vi "Continue Z Scan.vi"(7 "Error Signal Notifier":refnum<notifier>, 8 "error in (no error)":errorcluster, 9 "Automation State In":T1, 10 "Automation Queue":refnum<queue>, 11 "UI Queue":refnum<queue>) -> (0 "error out":errorcluster, 1 "Automation State Out":T1, 2 "Keep looping?":bool)   [LabVIEW 2013, in "Automation.lvlib"]
uses:
  Automation.lvlib
  Automation State.ctl
  Zscan Settings.ctl
  support/Message Queue/Message Cluster.ctl
  Feedback/Error Signal.ctl
  support/Message Queue/Enqueue Message (Single).vi
  support/Message Queue/Message Queue.lvlib
  Feedback/Feedback.lvlib
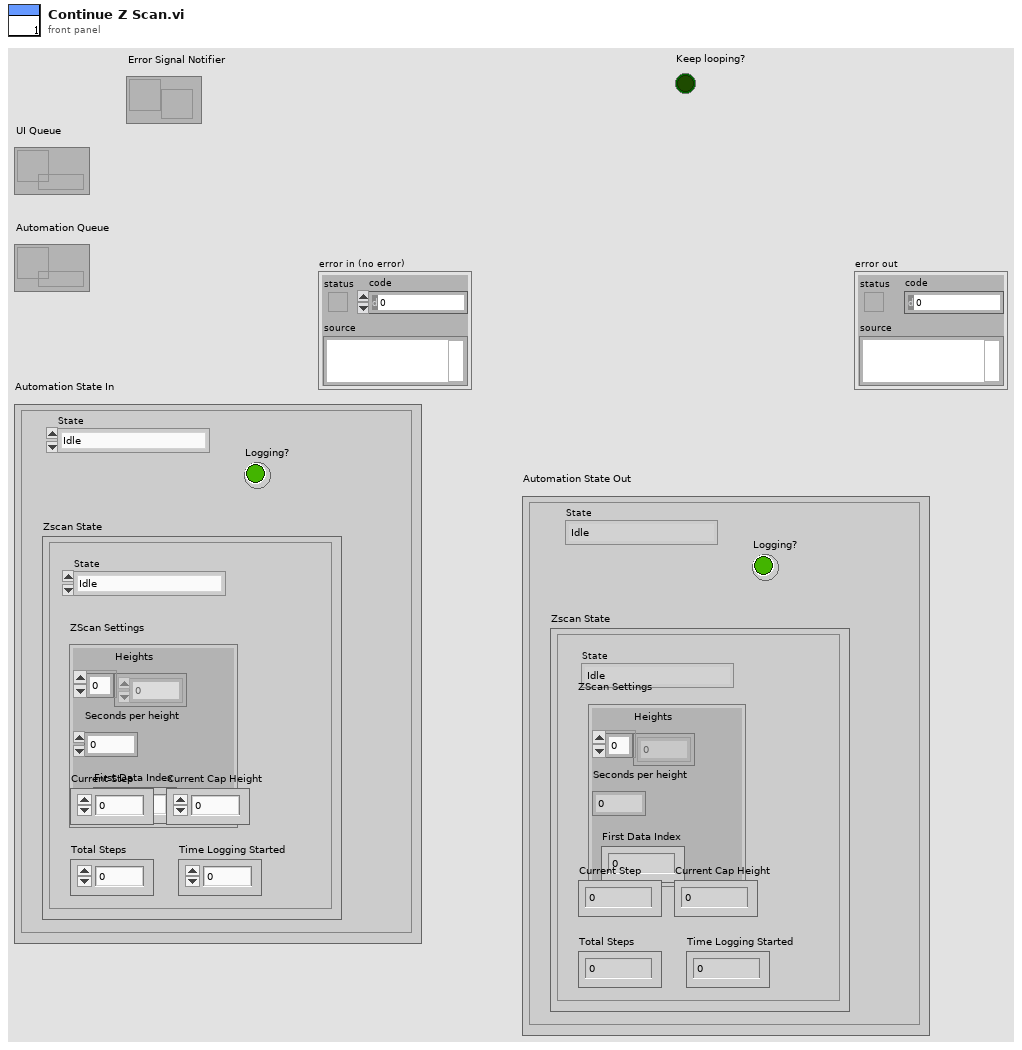
[diagram p1: front panel]
types:
  T1 = typedef "Automation.lvlib/Automation State.ctl" = cluster{"State":enum16{"Idle", "Zscan"}, "Logging?":bool, "Zscan State":cluster{"State":enum16{"Idle", "Waiting for lock", "Waiting for acquisition"}, "ZScan Settings":T2, "Current Step":i32, "Current Cap Height":dbl, "Total Steps":i32, "Time Logging Started":dbl}}
  T2 = typedef "Automation.lvlib/Zscan Settings.ctl" = cluster{"Heights":dbl[], "Seconds per height":i32, "First Data Index":i32}
  T3 = cluster{"State":enum16{"Idle", "Waiting for lock", "Waiting for acquisition"}, "ZScan Settings":T2, "Current Step":i32, "Current Cap Height":dbl, "Total Steps":i32, "Time Logging Started":dbl}
  T4 = enum16{"Idle", "Waiting for lock", "Waiting for acquisition"}
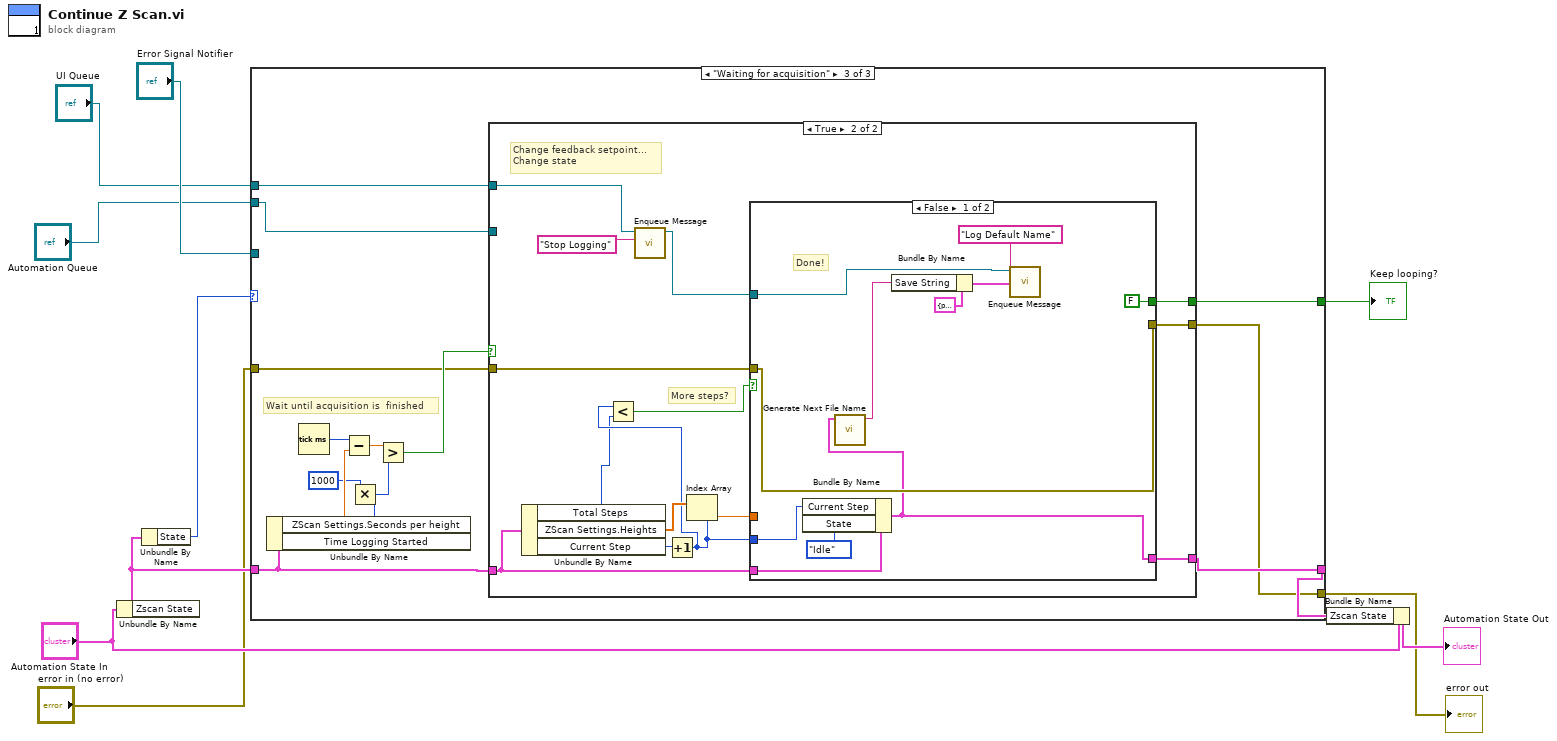
[diagram p0: block diagram]
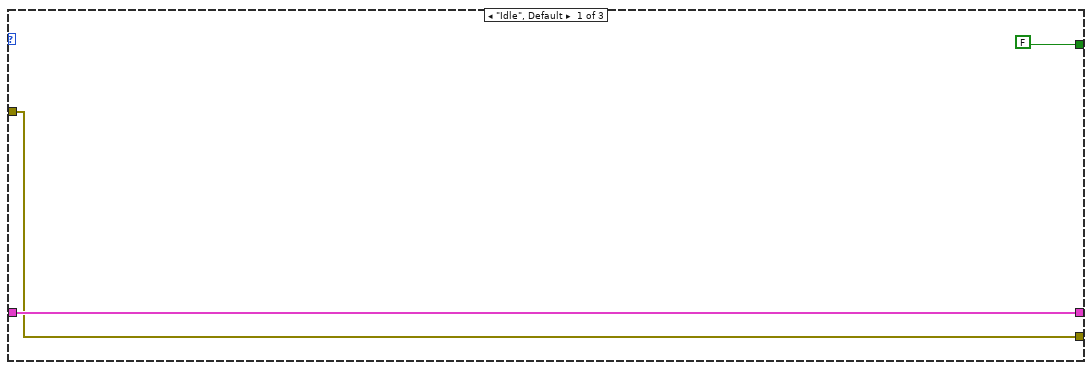
[diagram p2: hidden frame]
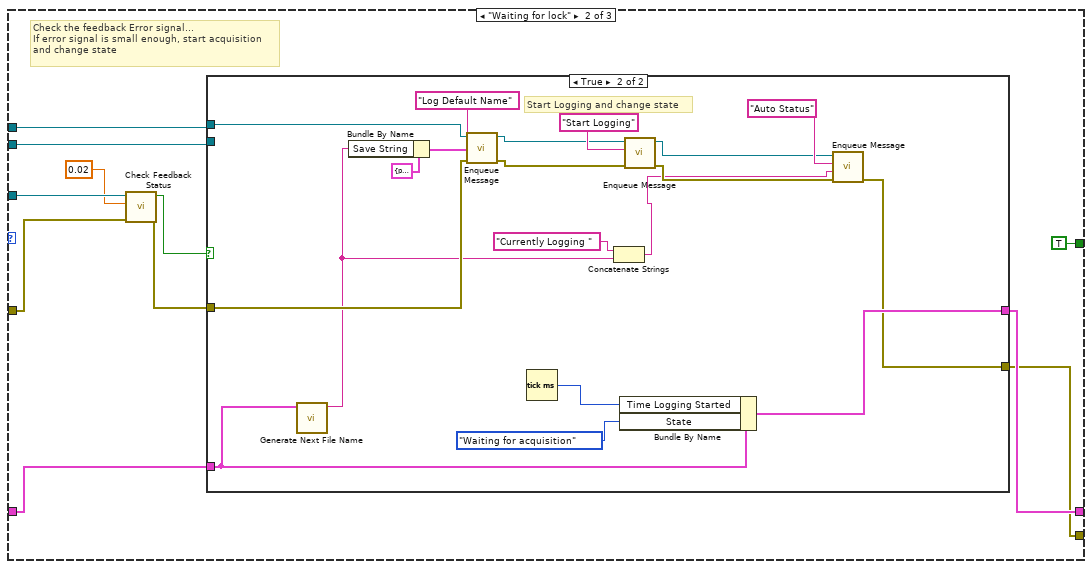
[diagram p3: hidden frame]
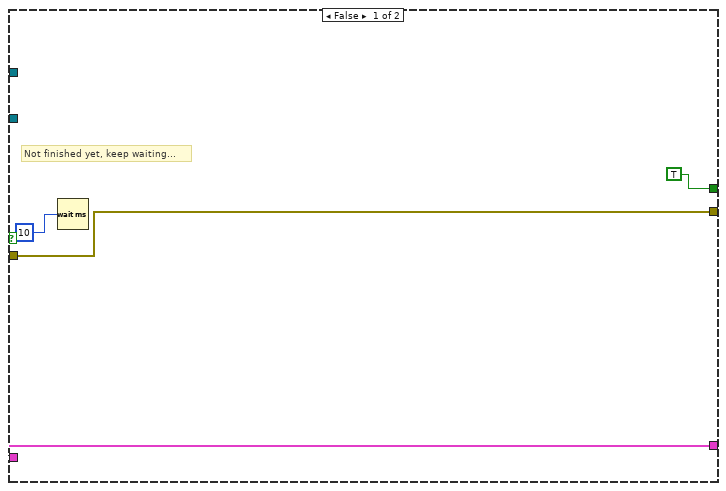
[diagram p5: hidden frame]
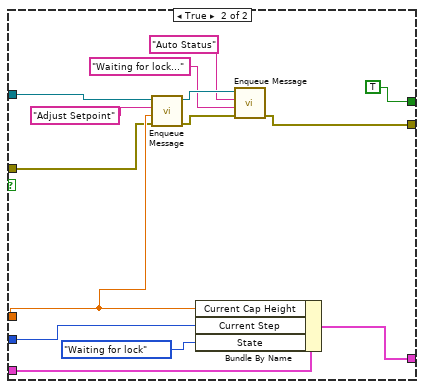
[diagram p6: hidden frame]
diagram:
  n1 = Unbundle By Name("Automation State In") -> ("Zscan State"=w8:T3)
  n2 = Unbundle By Name(w8) -> ("State"=w7:T4)
  n3 = case shown="\"Waiting for acquisition\"" w7 {
    tunnel: [w14 w21 w52] -> w9
    tunnel: w8 -> [w14 w22 w53]
    tunnel: "Error Signal Notifier" -> [_ w25 _]
    tunnel: "Automation Queue" -> [_ w20 w48]
    tunnel: "error in (no error)" -> [w13 w16 w50]
    tunnel: [w13 w19 w49] -> w3
    tunnel: "UI Queue" -> [_ w17 w51]
    tunnel: [FALSE ("Keep looping?") TRUE ("Keep looping?") w47] -> w1
    frame "Idle", Default {
    }
    frame "Waiting for lock" {
      # "Check the feedback Error signal...\nIf error signal is small enough, start acquisition\nand change state"
      n4 = call "Check Feedback Status.vi"("error in (no error)"=w16, "Threshold (um)"=0.02, "Error Signal Notifier"=w25) -> ("error out"=w15:errorcluster, "Locked"=w23:bool)  [unwired: 7 in]
      n5 = case shown="True" w23 {
        tunnel: w22 -> [w27 w32]
        tunnel: [w27 w46] -> w21
        tunnel: w20 -> [_ _]
        tunnel: w15 -> [w26 w35]
        tunnel: [w26 w40] -> w19
        tunnel: w17 -> [_ w28]
        frame False {
          # "If not locked, keep looping"
        }
        frame True {
          # "Start Logging and change state"
          n6 = call "Generate Next File Name.vi"("Zscan State"=w32) -> ("String"=w30:string)  [unwired: 10 in]
          n7 = Bundle By Name(cluster=cluster{"Save Path":path, "Save String":string} {"Save Path"=path "", "Save String"=""} ("output cluster"), "Save String"=w30) -> (w33:cluster{"Save Path":path, "Save String":string})
          n8 = call-poly "Enqueue Message.vi"("error in (no error)"=w35, "Message Data"=w33, "Message"="Log Default Name", "Message Queue"=w28) -> ("error out"=w37:errorcluster, "dup Message Queue"=w36:refnum<queue>)  [unwired: 6 in]
          n9 = Tick Count (ms)() -> (millisecond timer value=w43:u32)
          n10 = Concatenate Strings("Currently Logging " ("Message"), w30) -> (w29:string)
          n11 = Bundle By Name(cluster=w32, "Time Logging Started"=w43, "State"=T4."Waiting for acquisition") -> (w46:T3)
          n12 = call-poly "Enqueue Message.vi"("error in (no error)"=w37, "Message"="Start Logging", "Message Queue"=w36) -> ("error out"=w41:errorcluster, "dup Message Queue"=w39:refnum<queue>)  [unwired: 7 in]
          n13 = call-poly "Enqueue Message.vi"("error in (no error)"=w41, "Message Data"=w29, "Message"="Auto Status", "Message Queue"=w39) -> ("error out"=w40:errorcluster)  [unwired: 6 in, 1 out]
        }
      }
    }
    frame "Waiting for acquisition" {
      # "Wait until acquisition is  finished"
      n14 = Unbundle By Name(w53) -> ("ZScan Settings.Seconds per height"=w57:i32, "Time Logging Started"=w59:dbl)
      n15 = Tick Count (ms)() -> (millisecond timer value=w60:u32)
      n16 = Subtract(x=w60, y=w59) -> (x-y=w58:dbl)
      n17 = Multiply(x=1000, y=w57) -> (x*y=w55:i32)
      n18 = Greater?(x=w58, y=w55) -> (0:w54:bool)
      n19 = case shown="True" w54 {
        tunnel: w53 -> [w63 w77]
        tunnel: [w63 w78] -> w52
        tunnel: w51 -> [_ w66]
        tunnel: w50 -> [w62 w73]
        tunnel: [w62 w72] -> w49
        tunnel: w48 -> [_ _]
        tunnel: [TRUE ("Keep looping?") w67] -> w47
        frame False {
          # "Not finished yet, keep waiting..."
          n20 = Wait (ms)(milliseconds to wait=u32 10) -> ()  [unwired: 1 out]
        }
        frame True {
          # "More steps?"
          # "Change feedback setpoint...\nChange state"
          n21 = Unbundle By Name(w77) -> ("Total Steps"=w70:i32, "ZScan Settings.Heights"=w75:dbl[], "Current Step"=w76:i32)
          n22 = call-poly "Enqueue Message.vi"("Message"="Stop Logging", "Message Queue"=w66) -> ("dup Message Queue"=w65:refnum<queue>)  [unwired: 8 in, 1 out]
          n23 = Increment(x=w76) -> (x+1=w71:i32)
          n24 = Less?(x=w71, y=w70) -> (x < y?=w69:bool)
          n25 = Index Array(array=w75, index=w71) -> (element=w74:dbl)
          n26 = case shown="False" w69 {
            tunnel: [w79 w102] -> w78
            tunnel: w77 -> [w87 w101]
            tunnel: w71 -> [w80 w100]
            tunnel: w65 -> [w82 w98]
            tunnel: w74 -> [_ w97]
            tunnel: w73 -> [w89 w96]
            tunnel: [w89 w92] -> w72
            tunnel: [FALSE ("Keep looping?") TRUE ("Keep looping?")] -> w67
            frame False {
              # "Done!"
              n27 = Bundle By Name(cluster=w87, "Current Step"=w80, "State"=T4."Idle") -> (w79:T3)
              n28 = call "Generate Next File Name.vi"("Zscan State"=w79) -> ("String"=w81:string)  [unwired: 10 in]
              n29 = Bundle By Name(cluster=cluster{"Save Path":path, "Save String":string} {"Save Path"=path "", "Save String"=""} ("output cluster"), "Save String"=w81) -> (w83:cluster{"Save Path":path, "Save String":string})
              n30 = call-poly "Enqueue Message.vi"("Message Data"=w83, "Message"="Log Default Name", "Message Queue"=w82) -> ()  [unwired: 7 in, 2 out]
            }
            frame True {
              n31 = call-poly "Enqueue Message.vi"("error in (no error)"=w96, "Message Data"=w97, "Message"="Adjust Setpoint", "Message Queue"=w98) -> ("error out"=w93:errorcluster, "dup Message Queue"=w94:refnum<queue>)  [unwired: 6 in]
              n32 = Bundle By Name(cluster=w101, "Current Cap Height"=w97, "Current Step"=w100, "State"=T4."Waiting for lock") -> (w102:T3)
              n33 = call-poly "Enqueue Message.vi"("error in (no error)"=w93, "Message Data"="Waiting for lock..." ("Message"), "Message"="Auto Status", "Message Queue"=w94) -> ("error out"=w92:errorcluster)  [unwired: 6 in, 1 out]
            }
          }
        }
      }
    }
  }
  "error out" <- w3
  "Keep looping?" <- w1
  n34 = Bundle By Name(cluster="Automation State In", "Zscan State"=w9) -> (→"Automation State Out":T1)
